vi "APD.vi"() -> ()   [LabVIEW 2013]
panel:
  in  "Exposure Time [ms]":i32 min=1
  out "Waveform Chart":cluster{"Numeric":i32, "Numeric":i32}[](graph)
  in  "Channel 0":i32
  in  "Channel 1":i32
  out "number":u32
  in  "Array":bool[](array[boolean])
  in  "stop":bool
  out "Error Out":errorcluster
  in  "Device ID":i32
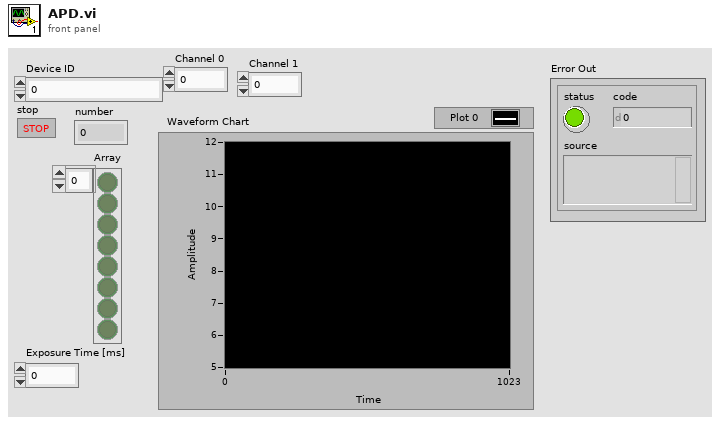
[diagram p1: front panel]
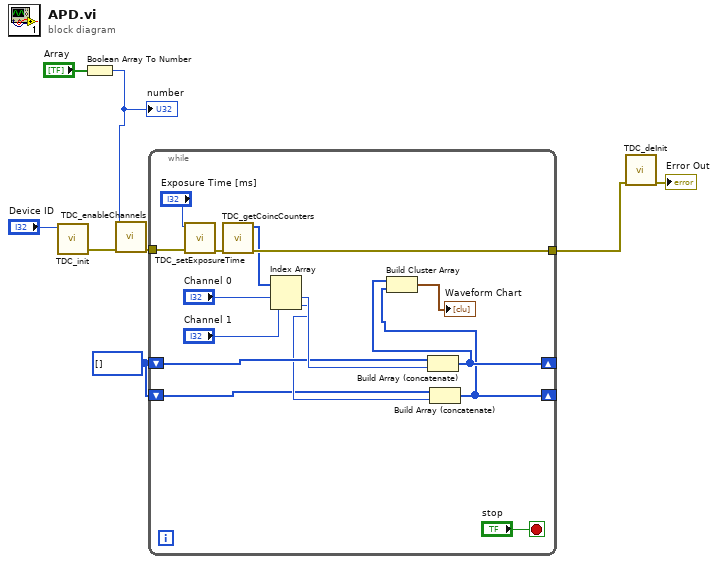
[diagram p0: block diagram]
diagram:
  w1 = i32[] []
  n1 = call "TDC_init.vi"("Device ID"="Device ID") -> ("Error Out"=w5:errorcluster)  [unwired: 10 in]
  n2 = Boolean Array To Number(Boolean array="Array") -> (number=w2:u32)
  "number" <- w2
  n3 = call "TDC_enableChannels.vi"("Error In"=w5, "channelMask"=w2) -> ("Error Out"=w4:errorcluster)  [unwired: 9 in]
  n4 = while {
    tunnel: [w22] -> w7
    tunnel: w4 -> [w11]
    shift-right: [w14] -> _
    shift-left: w1 -> [w17]
    shift-right: [w13] -> _
    shift-left: w1 -> [w15]
    stop <- "stop" stop-if-true
    n5 = call "TDC_setExposureTime.vi"("Error In"=w11, "Exposure Time [ms]"="Exposure Time [ms]") -> ("Error Out"=w10:errorcluster)  [unwired: 9 in]
    n6 = call "TDC_getCoincCounters.vi"("Error In"=w10) -> ("Error Out"=w22:errorcluster, "Coincidence Counters"=w21:i32[])  [unwired: 9 in]
    n7 = Index Array(array=w21, index #1="Channel 0", index #2="Channel 1") -> (element #1=w18:i32, element #2=w16:i32)
    n8 = Build Array (concatenate)(w17, w18) -> (w14:i32[])
    n9 = Build Array (concatenate)(w15, w16) -> (w13:i32[])
    n10 = Build Cluster Array(w14, w13) -> (→"Waveform Chart":cluster{"Numeric":i32, "Numeric":i32}[])
  }
  n11 = call "TDC_deInit.vi"("Error In"=w7) -> ("Error Out"=→"Error Out":errorcluster)  [unwired: 10 in]
